vi "robot change attitude.vi"(8 "error in (no error)":errorcluster, 10 "float speed":sgl, 11 "robot_id":i32) -> (0 "error out":errorcluster)   [LabVIEW 2020]
uses:
  small_scara_interface.dll
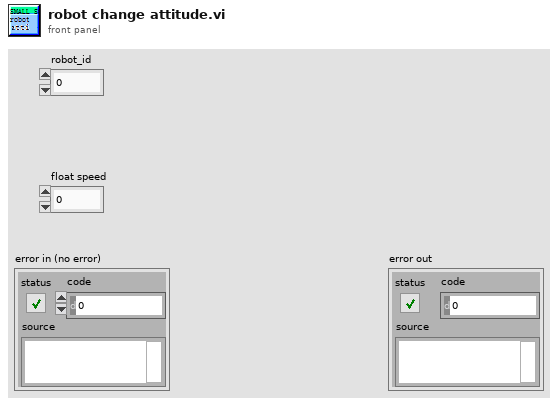
[diagram p1: front panel]
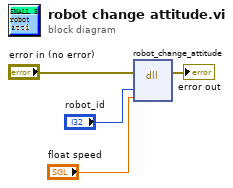
[diagram p0: block diagram]
diagram:
  n1 = dll-call lib="C:/Users/15239/Desktop/AutoChem_test/subvi/robot/subvi/Robot-HL/small_scara_interface/small_scara_interface.*" fn="robot_change_attitude"(error in="error in (no error)", "robot_id"="robot_id", "float speed"="float speed") -> (error out=→"error out":errorcluster)  [unwired: 5 in, 1 out]
